vi "Set NotifyIcon Icon.vi"(4 "error in (no error)":errorcluster, 6 "Icon path":path, 7 "NotifyIcon":refnum<k24>) -> (0 "error out":errorcluster, 3 "NotifyIcon Out":refnum<k24>)   [LabVIEW 2014, in "NotifyIcon.lvlib"]
uses:
  NotifyIcon.lvlib
  System.Windows.Forms
  System.Drawing
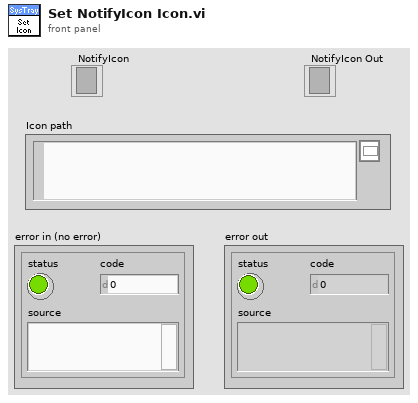
[diagram p1: front panel]
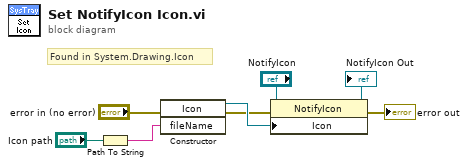
[diagram p0: block diagram]
diagram:
  # "Found in System.Drawing.Icon"
  n1 = Path To String(path="Icon path") -> (string=w7:string)
  n2 = constructor class="Icon"(error in="error in (no error)", "fileName"=w7) -> (reference out=w6:refnum<k24>, error out=w5:errorcluster)  [unwired: 2 in, 2 out]
  n3 = property class="NotifyIcon"(reference="NotifyIcon", error in=w5, "Icon"=w6) -> (reference out=→"NotifyIcon Out":refnum<k24>, error out=→"error out":errorcluster)
